vi "Write Capacity Unit (Standard Volume Flow).vi"(8 "error in":errorcluster, 10 "Standard Volue Flow":T1 items=["uls/h", "uls/min", "uls/s", "mls/h", "mls/min", "mls/s", "ls/h", "ls/min", "ls/s", "ccs/h", "ccn/min", "ccs/s", "mm3s/h", "mm3s/m", "mm3s/s", "cm3s/h", "cm3s/m", "cm3s/s", "m3s/h", "m3s/min", "m3s/s"], 11 "MB_TCP session in":refnum<class "MB_Master_TCP.lvclass">) -> (0 "error out":errorcluster, 2 "Capacity Unit":string, 3 "MB session out":refnum<class "MB_Master_TCP.lvclass">)   [LabVIEW 2024, in "Bronkhorst Flexi-Flow ModbusTCP API.lvlib"]
uses:
  Modbus Flexi-Flow API/Bronkhorst Flexi-Flow ModbusTCP API.lvlib
  Modbus Flexi-Flow API/Write String Register.vi
  Modbus Flexi-Flow API/Read String Register.vi
  Modbus Flexi-Flow API/PDU Address String Params--ring.ctl
  <userlib>/_OpenG.lib/string/string.llb/openg_string.lvlib
  <vilib>/Plasmionique/MB Master/MB_Master_TCP/MB_Master_TCP.lvclass
  Modbus Flexi-Flow API/Capacity Units (Standard Volume Flow).ctl
panel:
  # "ug/h, ug/min, ug/s,\nmg/h, mg/min, mg/s,\ng/h, g/min, g/s,\nkg/h, kg/min, kg/s"
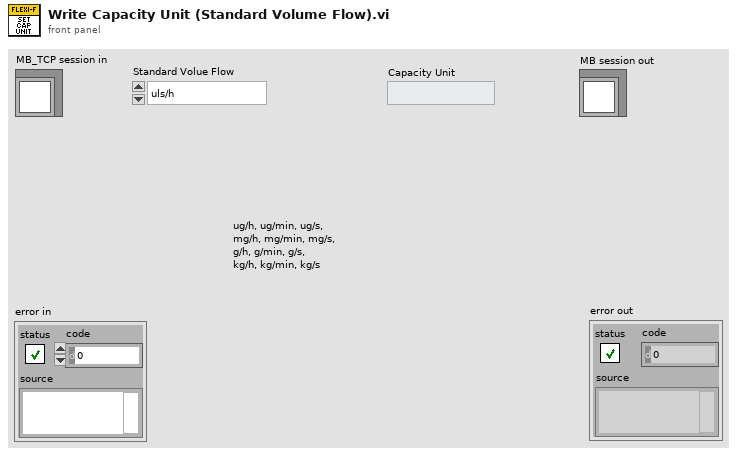
[diagram p1: front panel]
types:
  T1 = typedef "Bronkhorst Flexi-Flow ModbusTCP API.lvlib/Capacity Units (Standard Volume Flow).ctl" = u16
  T2 = typedef "Bronkhorst Flexi-Flow ModbusTCP API.lvlib/PDU Address String Params--ring.ctl" = u16
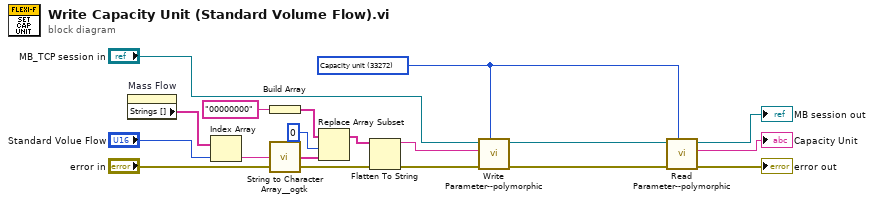
[diagram p0: block diagram]
diagram:
  w13 = T2 33272 items=["Fluid name"=33160, "Capacity unit"=33272, "User tag"=61744] ("PDU Address String Params")
  n1 = property on="Mass Flow" class="Ring (strict)"() -> ("Strings []"=w12:string[])  [unwired: 2 in, 2 out]
  n2 = Index Array(array=w12, index="Standard Volue Flow") -> (element=w9:string)
  n3 = Build Array("00000000") -> (w7:string[])
  n4 = call <userlib>:"String to Character Array__ogtk.vi"("Input String"=w9) -> ("Character Array"=w6:string[])
  n5 = Replace Array Subset(array=w7, new element=w6, index=0) -> (w4:string[])
  n6 = Flatten To String(anything=w4, error in (no error)="error in") -> (data string=w3:string, error out=w1:errorcluster)  [unwired: 2 in, 1 out]
  n7 = call-poly "Write Parameter--polymorphic.vi"("PDU Address String Params"=w13, "error in"=w1, "String"=w3, "MB_TCP session in"="MB_TCP session in") -> ("error out"=w15:errorcluster, "MB session out"=w17:refnum<class "MB_Master_TCP.lvclass">)  [unwired: 6 in]
  n8 = call-poly "Read Parameter--polymorphic.vi"("PDU Address String Params"=w13, "error in"=w15, "MB_TCP session in"=w17) -> ("error out"=→"error out":errorcluster, "Value"=→"Capacity Unit":string, "MB session out"=→"MB session out":refnum<class "MB_Master_TCP.lvclass">)  [unwired: 6 in]
